vi "Part 1.vi"(11 "Input":string) -> (3 "Output":i64)   [LabVIEW 2021]
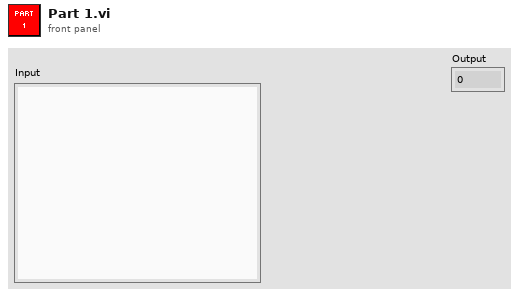
[diagram p1: front panel]
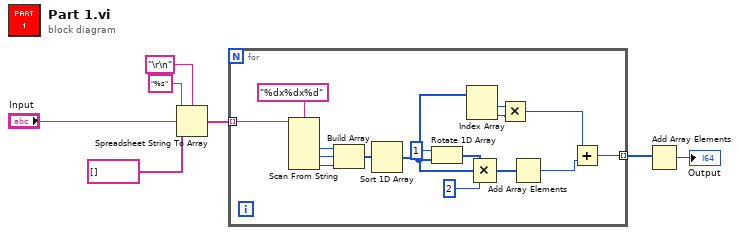
[diagram p0: block diagram]
diagram:
  n1 = Spreadsheet String To Array(delimiter (Tab)="\r\n", format string="%s", spreadsheet string="Input", array type (2D Dbl)=string[] []) -> (array=w3:string[])
  n2 = for {
    tunnel: w3 -> [w23] mode=indexing
    tunnel: [w10] -> w2 mode=indexing
    n3 = Scan From String(format string="%dx%dx%d", input string=w23) -> (output 1=w21:i32, output 2=w20:i32, output 3=w19:i32)  [unwired: 5 in, 3 out]
    n4 = Build Array(w21, w20, w19) -> (w18:i32[])
    n5 = Sort 1D Array(array=w18) -> (sorted array=w15:i32[])
    n6 = Rotate 1D Array(1:w15, 2:1 ("n")) -> (0:w16:i32[])
    n7 = Index Array(array=w15) -> (element #1=w13:i32, element #2=w14:i32)  [unwired: 2 in]
    n8 = Compound Arithmetic op=MULTIPLY(w16, w15, 2 ("n")) -> (w12:i32[])
    n9 = Multiply(x=w13, y=w14) -> (x*y=w11:i32)
    n10 = Add Array Elements(numeric array=w12) -> (sum=w9:i32)
    n11 = Add(x=w11, y=w9) -> (x+y=w10:i32)
  }
  n12 = Add Array Elements(numeric array=w2) -> (sum=→"Output":i32)
